vi "mod_FSK Transmitter.vi"(0 "Symbol Rate, Hz":dbl=1.0 format="%.2f", 1 "Reset?":bool, 2 "# Samples per Symbol":i32=16, 5 "FSK Specific":T1={"M-FSK"=2, "FSK deviation (Hz)"=3000.0, "Symbol Phase Continuity"=enum."continuous"} {"FSK deviation (Hz)" format="%.2f"; "M-FSK" min=2 step=2}, 7 "Message":T3={"# Guard Bits"=2, "# Sync Bits"=20, "# Message Bits"=1000, "PN sequence order"=9}, 9 "System Filter":T2={"TX Filter"=enum."Gaussian", "BT"=0.5, "filter length"=20} {"BT" format="%.2f"}, 11 "error in (no error)":errorcluster) -> (4 "Output Complex Waveform":T6 {"Y" format="%.3f"; "dt" format="%^.2e"; "t0" format="%.4f"}, 6 "Signal Description":T5 {"FSK system parameters"."symbol map" format="%.2f"; "matched filter coefficients" format="%.2f"; "pulse shaping filter coefficients" format="%.2f"; "Sync (Symbols)" format="%.2f"}, 15 "error out":errorcluster)   [LabVIEW 2020, in "niDMT.lvlib"]
doc: "This example demonstrates generation of a FSK-modulated signal. You can specify characteristics of the message signal such as PN sequence order, number of guard bits, number of sync bits, and transmit filter parameters. You can extend this example to download the generated FSK signal to GPIB-based RF signal generators."
uses:
  <vilib>/addons/Modulation/niDMT.lvlib
  <vilib>/addons/Modulation/Digital/Support/Controls/FSK System Parameters.ctl
  <vilib>/addons/Modulation/Analog/controls/Complex Data Waveform.ctl
  <vilib>/addons/Modulation/Analog/support/mod_Set Error Source.vi
  <vilib>/addons/Modulation/Digital/Support/Common/Validators/mod_Generate Filter Coefficients Validate.vi
  <vilib>/addons/Modulation/Digital/General/subVIs/mod_Generate Filter Coefficients.vi
  <vilib>/addons/Modulation/Digital/General/MT Generate FSK System Parameters(M).vi
  <vilib>/addons/Modulation/niAMT.lvlib
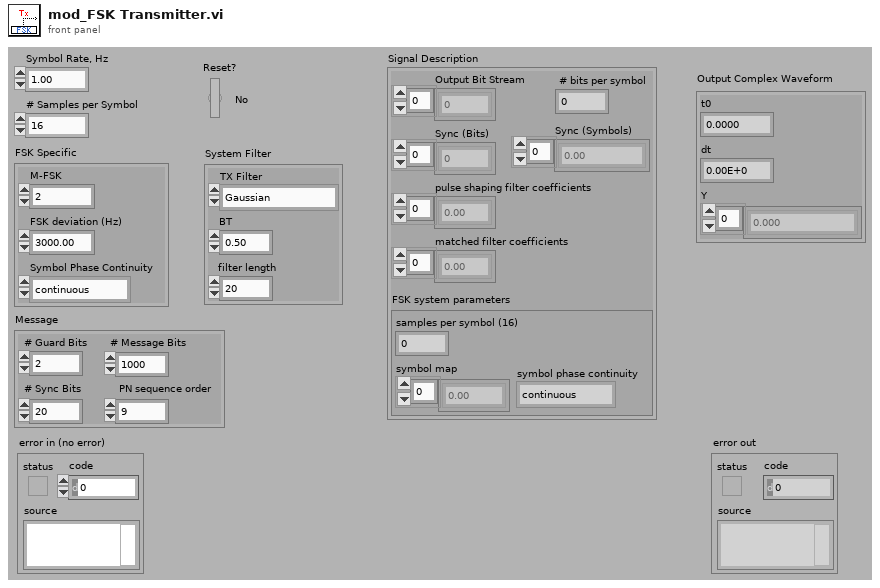
[diagram p1: front panel]
types:
  T1 = cluster{"M-FSK":i32, "FSK deviation (Hz)":dbl, "Symbol Phase Continuity":enum16{"continuous", "discontinuous"}}
  T2 = cluster{"TX Filter":enum16{"none", "Raised Cosine", "Root Raised Cos", "Gaussian"}, "BT":dbl, "filter length":i32}
  T3 = cluster{"# Guard Bits":i32, "# Sync Bits":i32, "# Message Bits":i32, "PN sequence order":i32}
  T4 = typedef "niDMT.lvlib/FSK System Parameters.ctl" = cluster{"samples per symbol (16)":i32, "symbol map":dbl[], "symbol phase continuity":enum16{"continuous", "discontinuous"}}
  T5 = cluster{"Output Bit Stream":i8[], " # bits per symbol":i32, "Sync (Bits)":i8[], "Sync (Symbols)":cdb[], "pulse shaping filter coefficients":dbl[], "matched filter coefficients":dbl[], "FSK system parameters":T4}
  T6 = typedef "niAMT.lvlib/Complex Data Waveform.ctl" = cluster{"t0":dbl, "dt":dbl, "Y":cdb[]}
  T7 = cluster{"Output Bit Stream":i8[], "# bits per symbol":i32, "Sync (Bits)":i8[], "Sync (Symbols)":cdb[], "pulse shaping filter coefficients":dbl[], "matched filter coefficients":dbl[], "FSK system parameters":T4}
  T8 = enum16{"none", "Raised Cosine", "Root Raised Cos", "Gaussian"}
  T9 = cluster{"samples per symbol (16)":i32, "symbol map":dbl[], "symbol phase continuity":enum16{"continuous", "discontinuous"}}
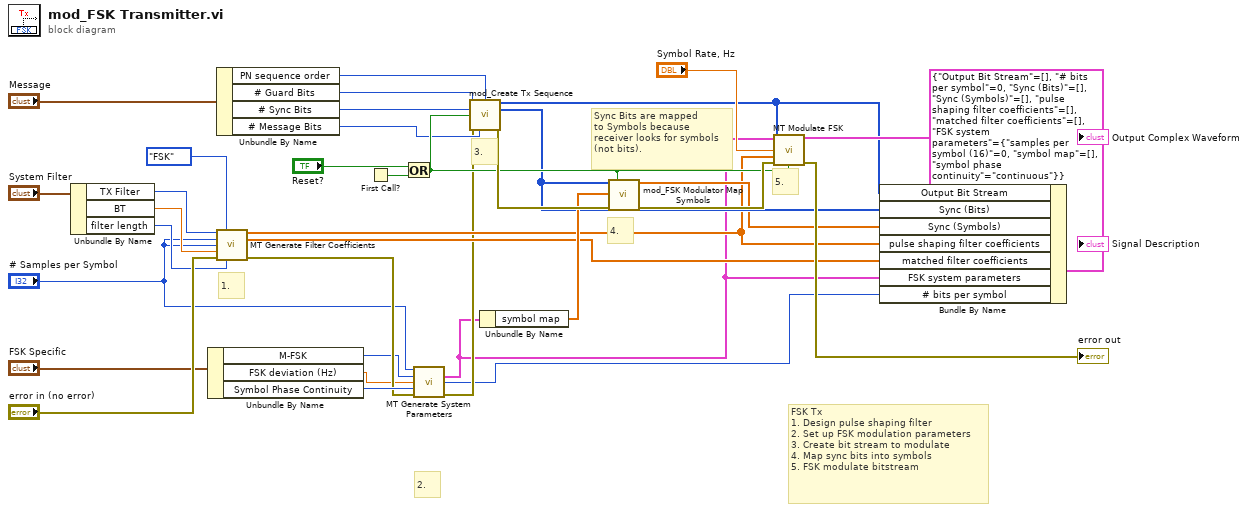
[diagram p0: block diagram]
diagram:
  # "5."
  # "4."
  # "2."
  # "3."
  # "1."
  # "FSK Tx\n1. Design pulse shaping filter\n2. Set up FSK modulation parameters\n3. Create bit stream to modulate\n4. Map sync bits into symbols\n5. FSK modulate bitstream"
  # "Sync Bits are mapped\nto Symbols because\nreceiver looks for symbols\n(not bits)."
  n1 = Unbundle By Name("System Filter") -> ("TX Filter"=w21:T8, "BT"=w20:dbl, "filter length"=w19:i32)
  n2 = Unbundle By Name("FSK Specific") -> ("M-FSK"=w3:i32, "FSK deviation (Hz)"=w4:dbl, "Symbol Phase Continuity"=w6:enum16{"continuous", "discontinuous"})
  n3 = Unbundle By Name("Message") -> ("PN sequence order"=w10:i32, "# Guard Bits"=w25:i32, "# Sync Bits"=w24:i32, "# Message Bits"=w23:i32)
  n4 = call <vilib>:"MT Generate Filter Coefficients.vi"("pulse shaping filter (none)"=w21, "modulation type"=enum16{"FSK", "PSK", "QAM", "MSK", "PAM", "ASK"}."FSK", "pulse shaping samples per symbol (16)"="# Samples per Symbol", "matched samples per symbol (16)"="# Samples per Symbol", "filter parameter"=w20, "error in (no error)"="error in (no error)", "filter length (symbols)"=w19) -> ("pulse shaping filter coefficients"=w14:dbl[], "matched filter coefficients"=w13:dbl[], "error out"=w5:errorcluster)  [unwired: 6 out]
  n5 = First Call?() -> (First Call?: T/F=w30:bool)
  n6 = Or(x="Reset?", y=w30) -> (x .or. y?=w28:bool)
  n7 = call-poly <vilib>:"MT Generate System Parameters.vi"("samples per symbol (16)"="# Samples per Symbol", "M-FSK (2)"=w3, "FSK deviation (Hz)"=w4, "symbol phase continuity"=w6, "error in (no error)"=w5) -> ("FSK system parameters"=w8:T9, "bits per symbol"=w7:i32, "error out"=w9:errorcluster)  [unwired: 8 out]
  n8 = call <vilib>:"mod_Create Tx Sequence.vi"("# Guard Bits (2)"=w25, "PN sequence order (9)"=w10, "# Sync Bits (20)"=w24, "Reset? (T)"=w28, "error in (no error)"=w9, "# Message Bits"=w23) -> ("Output Bit Stream"=w17:i8[], "Last Sync Pattern"=w16:i8[], "error out"=w34:errorcluster)  [unwired: 3 in, 4 out]
  n9 = Unbundle By Name(w8) -> ("symbol map"=w27:dbl[])
  n10 = call <vilib>:"mod_FSK Modulator Map Symbols.vi"("Input Bit Stream"=w16, "Symbol Map"=w27, "error in (no error)"=w34, "Reset? (T)"=w28) -> ("Symbols Out"=w15:dbl[], "error out"=w35:errorcluster)  [unwired: 10 out]
  n11 = call <vilib>:"MT Modulate FSK.vi"("input bit stream"=w17, "FSK system parameters"=w8, "symbol rate (Hz)"="Symbol Rate, Hz", "pulse shaping filter coefficients"=w14, "error in (no error)"=w35, "reset? (T)"=w28) -> ("output complex waveform"=→"Output Complex Waveform":T6, "error out"=→"error out":errorcluster)  [unwired: 1 in, 7 out]
  n12 = Bundle By Name(cluster=T7 {"Output Bit Stream"=[], "# bits per symbol"=0, "Sync (Bits)"=[], "Sync (Symbols)"=[], "pulse shaping filter coefficients"=[], "matched filter coefficients"=[], "FSK system parameters"={"samples per symbol (16)"=0, "symbol map"=[], "symbol phase continuity"=enum."continuous"}} ("input cluster"), "Output Bit Stream"=w17, "Sync (Bits)"=w16, "Sync (Symbols)"=w15, "pulse shaping filter coefficients"=w14, "matched filter coefficients"=w13, "FSK system parameters"=w8, "# bits per symbol"=w7) -> (→"Signal Description":T7)
